vi "Get Number of Channels.vi"(8 "error in (no error)":errorcluster, 11 "Preview in":refnum<class "Preview.lvclass">) -> (0 "error out":errorcluster, 2 "size(s)":i32, 3 "Preview out":refnum<class "Preview.lvclass">)   [LabVIEW 2018, in "Preview Window.lvlib" / "Preview.lvclass"]
uses:
  Preview.lvclass
  Preview.lvclass/Preview.ctl
  Cfg Grandmaster/Class Chan Group/Read GroupChans.vi
  Measurements/Class Channel/Channel.lvclass
  Cfg Grandmaster/Class Chassis Cfg/ChassisCfg.lvclass
  Cfg Grandmaster/Class Chan Group/ChanGrp.lvclass
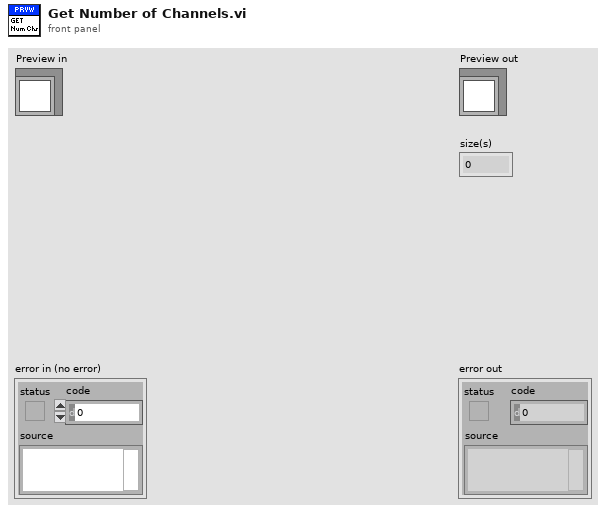
[diagram p1: front panel]
types:
  T1 = typedef "Selected Group.ctl" = cluster{"ChanGroup":i32, "Rate Class":T2}
  T2 = typedef "TE_Designator.ctl" = enum16{"High Speed", "Low Speed"}
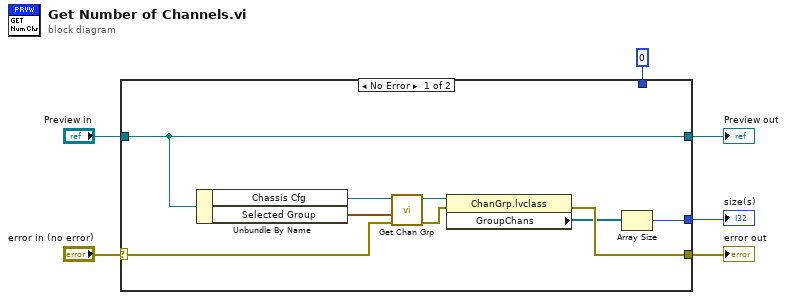
[diagram p0: block diagram]
diagram:
  n1 = case shown="No Error" "error in (no error)" {
    selector: "error in (no error)" -> [w11 w18]
    tunnel: [w10 w18] -> w5
    tunnel: [w9 w17] -> w3
    tunnel: "Preview in" -> [w9 w17]
    tunnel: [w7 w16] -> w2
    tunnel: 0 -> [_ w16]
    frame No Error {
      n2 = Unbundle By Name(w9) -> ("Chassis Cfg"=w15:refnum<class "ChassisCfg.lvclass">, "Selected Group"=w14:T1)
      n3 = call "Get Chan Grp.vi"("error in (no error)"=w11, "Selected Grp"=w14, "Chassis Cfg"=w15) -> ("error out"=w12:errorcluster, "Chan Group"=w13:refnum<class "ChanGrp.lvclass">)  [unwired: 7 in]
      n4 = property class="ChanGrp.lvclass"(reference=w13, error in=w12) -> (error out=w10:errorcluster, "GroupChans"=w8:refnum<class "Channel.lvclass">[])  [unwired: 1 out]
      n5 = Array Size(array=w8) -> (size(s)=w7:i32)
    }
    frame Error {
    }
  }
  "error out" <- w5
  "Preview out" <- w3
  "size(s)" <- w2
